vi "Humidity.vi"(1 "Humidity":dbl) -> (0 "Humidity Warning":bool)   [LabVIEW 2019]
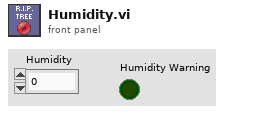
[diagram p1: front panel]
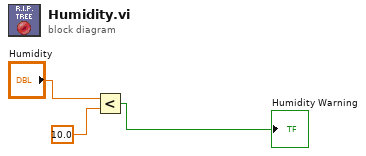
[diagram p0: block diagram]
diagram:
  n1 = Less?(x="Humidity", y=10.0) -> (x < y?=→"Humidity Warning":bool)
